vi "TIM101 Device Engine.vi"(0 "Unique Notifier Name":string, 11 "Serial Number":string[](array[string])) -> ()   [LabVIEW 2020]
uses:
  Actuators Controls/Actuators Note Type.ctl
  Actuators Controls/Actuators Actions.ctl
  TIM101 DLL/TIM101 Control.dll
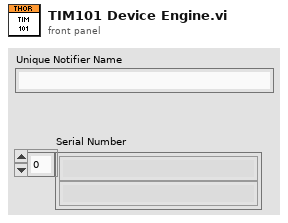
[diagram p1: front panel]
types:
  T1 = typedef "Actuators Note Type.ctl" = cluster{"Actions":T2, "Cmd Received ":bool, "Setpoint":dbl[], "Position":dbl[], "Axis":dbl}
  T2 = typedef "Actuators Actions.ctl" = enum16{"Nothing", "Get Position", "Move Absolute", "Move Relative", "Halt", "Quit"}
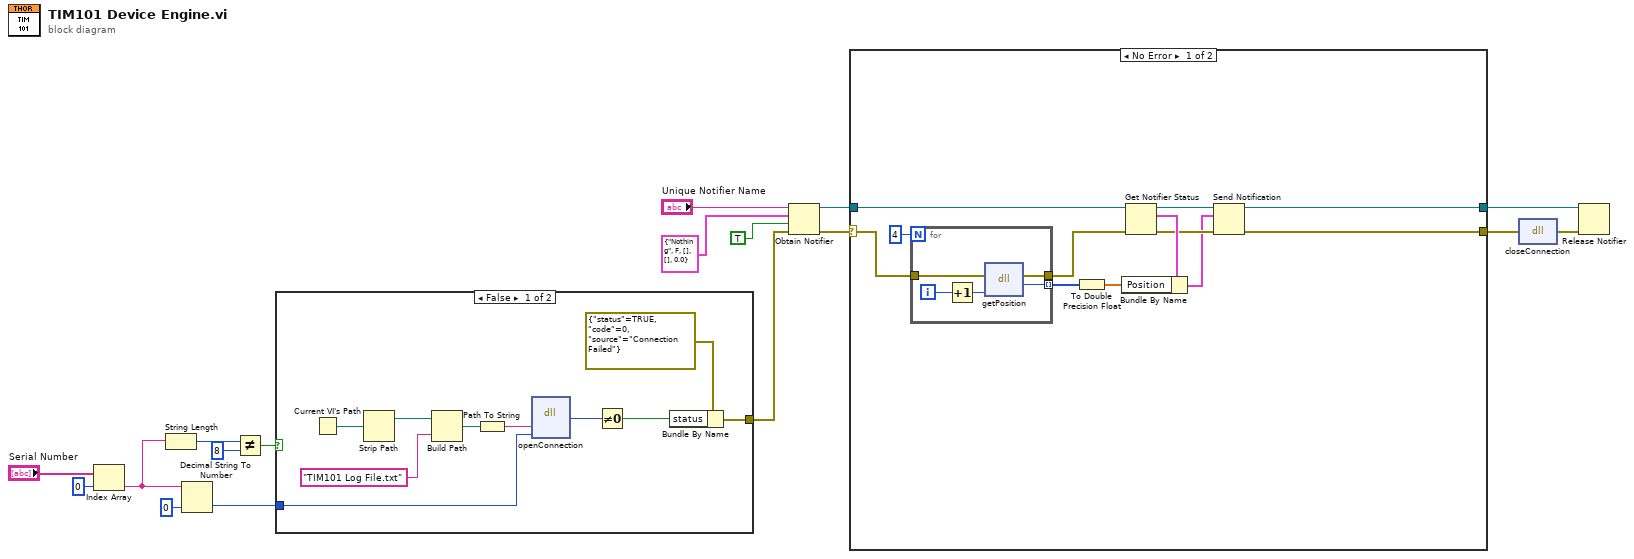
[diagram p0: block diagram]
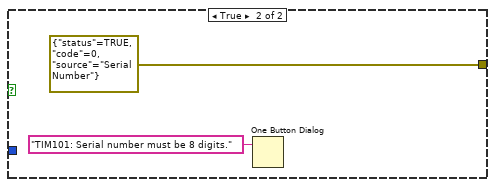
[diagram p3: hidden frame]
diagram:
  n1 = Index Array(array="Serial Number", index=0) -> (element=w14:string)
  n2 = String Length(string=w14) -> (length=w13:i32)
  n3 = Decimal String To Number(string=w14, default (0L)=0 ("default (0 I32)")) -> (number=w11:i32)  [unwired: 1 in, 1 out]
  n4 = Not Equal?(x=w13, y=8) -> (x != y?=w10:bool)
  n5 = case shown="False" w10 {
    tunnel: w11 -> [w18 _]
    tunnel: [w20 errorcluster {"status"=TRUE, "code"=0, "source"="Serial Number"} ("error out")] -> w6
    frame False {
      n6 = Current VI's Path() -> (path=w27:path)
      n7 = Strip Path(path=w27) -> (stripped path=w26:path)  [unwired: 1 out]
      n8 = Build Path(base path=w26, name or relative path="TIM101 Log File.txt") -> (appended path=w24:path)
      n9 = Path To String(path=w24) -> (string=w23:string)
      n10 = dll-call lib="C:/Users/user/Documents/Microscope-Control/Device Library/Actuators/Thorlabs/TIM101/TIM101 DLL/TIM101 Control.dll" fn="openConnection"("Log File"=w23, "Serial Number"=w18) -> ("Open Success"=w19:i32)  [unwired: 5 in, 2 out]
      n11 = Not Equal To 0?(x=w19) -> (x != 0?=w21:bool)
      n12 = Bundle By Name(cluster=errorcluster {"status"=TRUE, "code"=0, "source"="Connection Failed"} ("error out"), "status"=w21) -> (w20:errorcluster)
    }
    frame True {
      n13 = One Button Dialog(message="TIM101: Serial number must be 8 digits.") -> ()  [unwired: 1 in, 1 out]
    }
  }
  n14 = Obtain Notifier(name (unnamed)="Unique Notifier Name", notification data type=T1 {"Actions"=enum."Nothing", "Cmd Received "=FALSE, "Setpoint"=[], "Position"=[], "Axis"=0.0} ("Actuators Note"), create if not found? (T)=TRUE, error in (no error)=w6) -> (notifier out=w4:refnum<notifier>, error out=w5:errorcluster)  [unwired: 1 out]
  n15 = case shown="No Error" w5 {
    selector: w5 -> [w39 w47]
    tunnel: w4 -> [w38 w48]
    tunnel: [w31 w47] -> w3
    tunnel: [w30 w48] -> w2
    frame No Error {
      n16 = for {
        N: 4 -> [_]
        tunnel: w39 -> [w44]
        tunnel: [w43] -> w40 mode=indexing
        tunnel: [w42] -> w34
        i -> [w46]
        n17 = Increment(x=w46) -> (x+1=w45:i32)
        n18 = dll-call lib="C:/Users/user/Documents/Microscope-Control/Device Library/Actuators/Thorlabs/TIM101/TIM101 DLL/TIM101 Control.dll" fn="getPosition"(error in=w44, "Axis"=w45) -> (error out=w42:errorcluster, "Position"=w43:i32)  [unwired: 3 in, 1 out]
      }
      n19 = To Double Precision Float(number=w40) -> (double precision float=w36:dbl[])
      n20 = Get Notifier Status(notifier=w38, error in (no error)=w34) -> (notifier out=w35:refnum<notifier>, current notification=w37:T1, error out=w33:errorcluster)  [unwired: 2 out]
      n21 = Bundle By Name(cluster=w37, "Position"=w36) -> (w32:T1)
      n22 = Send Notification(notification=w32, notifier=w35, error in (no error)=w33) -> (notifier out=w30:refnum<notifier>, error out=w31:errorcluster)
    }
    frame Error {
    }
  }
  n23 = dll-call lib="C:/Users/user/Documents/Microscope-Control/Device Library/Actuators/Thorlabs/TIM101/TIM101 DLL/TIM101 Control.dll" fn="closeConnection"(error in=w3) -> (error out=w1:errorcluster)  [unwired: 3 in, 1 out]
  n24 = Release Notifier(notifier=w2, error in (no error)=w1) -> ()  [unwired: 1 in, 3 out]
